vi "Stages Messenger limit check.vi"(0 "Stage Notifier Name":string="ProScan3", 2 "Actions":T2, 5 "Setpoint":dbl[](array[numeric]), 7 "Axis":bool[](array[boolean]), 9 "Velocity":dbl, 11 "Misc":variant, 13 "Exit While Busy?":bool) -> (4 "Stage Notifier Name (Dup)":string, 6 "Positions":dbl[](array[numeric]), 8 "Status":T1, 15 "Error":errorcluster)   [LabVIEW 2021]
uses:
  Stages Controls/Stage Actions.ctl
  Stages Controls/Stage Status.ctl
  Stages Controls/Stage Notifier Element.ctl
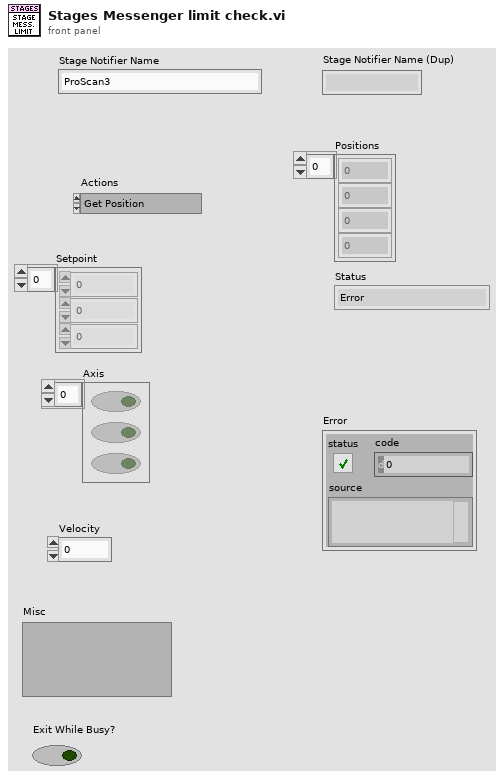
[diagram p1: front panel]
types:
  T1 = typedef "Stage Status.ctl" = enum16{"Error", "Abort", "Busy", "On Target"}
  T2 = typedef "Stage Actions.ctl" = enum16{"Get Position", "SERVO OFF", "SERVO ON", "SERVO ON/OFF", "MVR", "MOVE", "HALT", "ONTARGET", "ERROR", "REFERENCE", "INIT", "VELOCITY", "STATUS", "EXIT", "HOME", "ZEROPOS", "NANOPOS", "ANALOG", "QUIT"}
  T3 = typedef "Stage Notifier Element.ctl" = cluster{"Action":T2, "Axis":bool[], "Setpoint":dbl[], "Velocity":dbl, "Cmd Recvd?":bool, "Position":dbl[], "Status":T1, "Misc":variant, "Servo On?":bool}
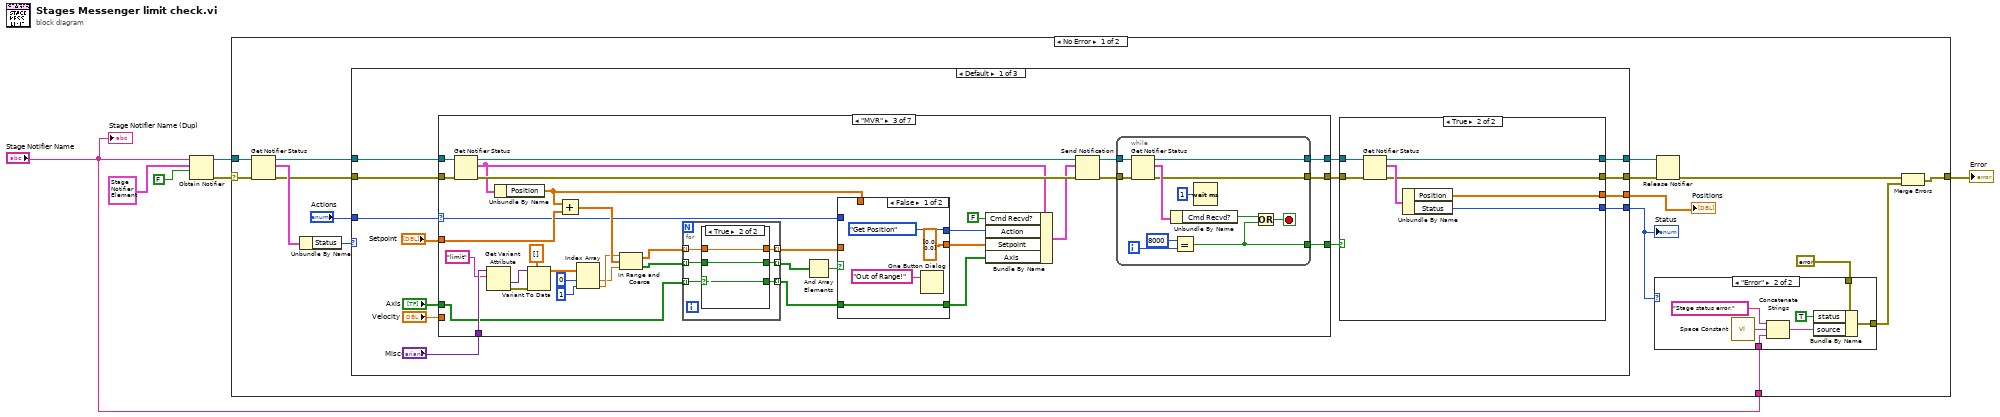
[diagram p0: block diagram]
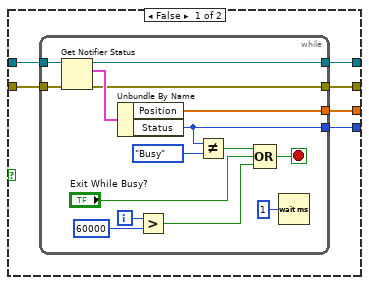
[diagram p3: hidden frame]
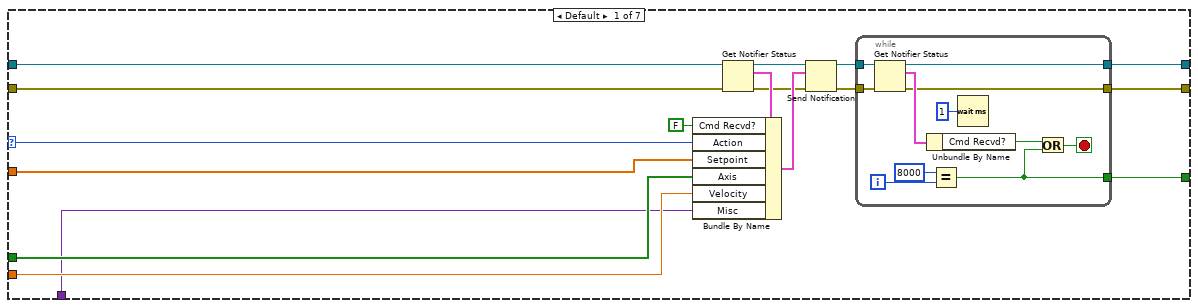
[diagram p4: hidden frame]
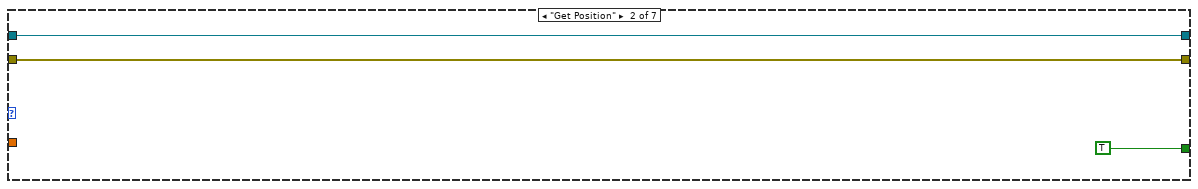
[diagram p5: hidden frame]
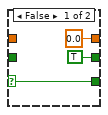
[diagram p6: hidden frame]
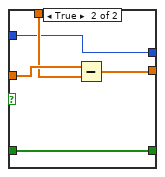
[diagram p7: hidden frame]
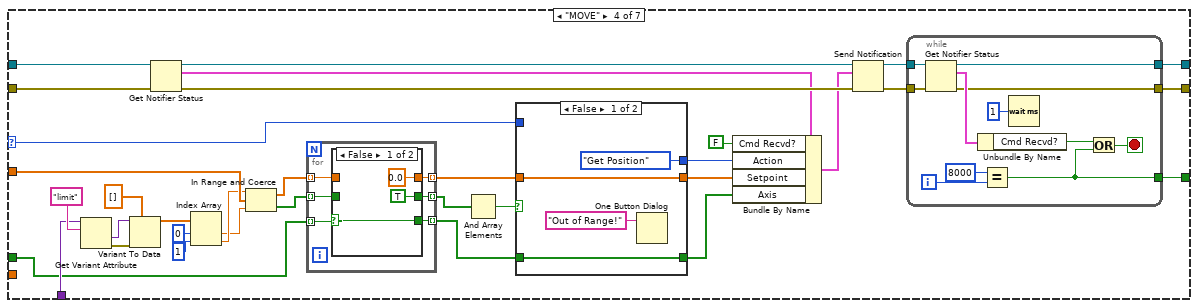
[diagram p8: hidden frame]
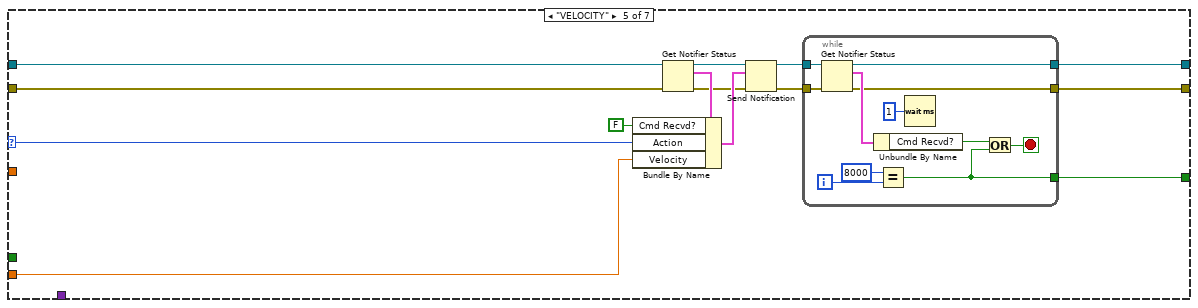
[diagram p11: hidden frame]
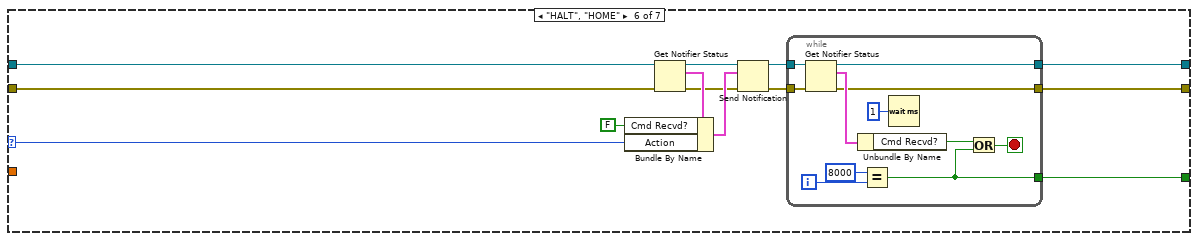
[diagram p12: hidden frame]
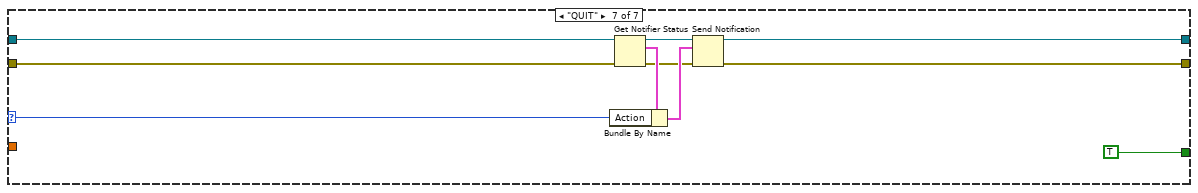
[diagram p13: hidden frame]
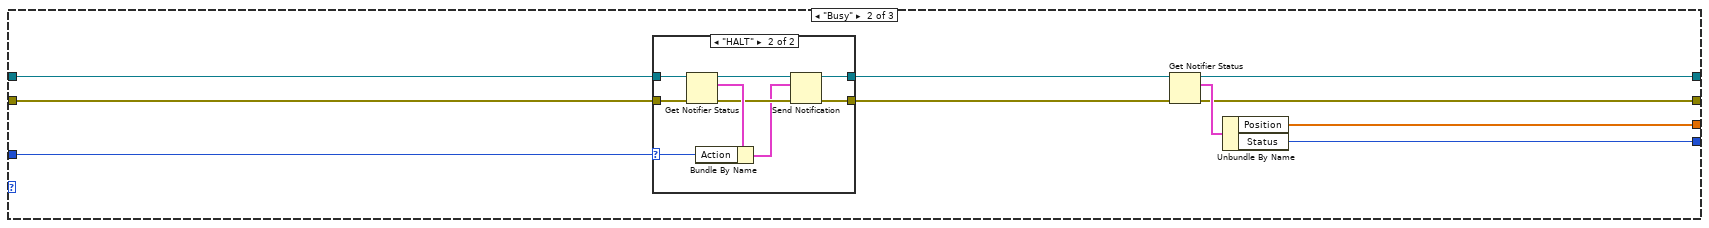
[diagram p14: hidden frame]
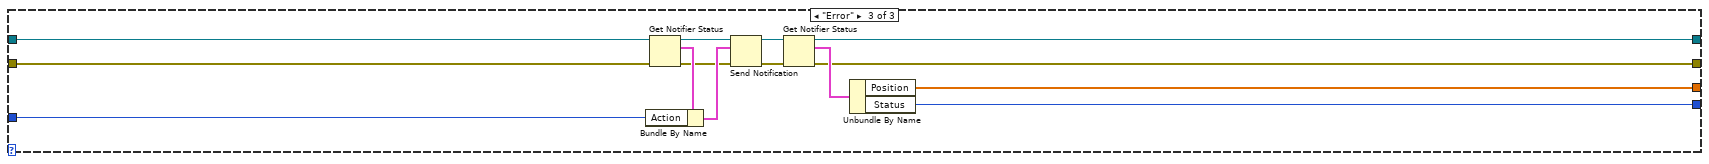
[diagram p16: hidden frame]
diagram:
  n1 = Obtain Notifier(name (unnamed)="Stage Notifier Name", notification data type=T3 {"Action"=enum."Get Position", "Axis"=[], "Setpoint"=[], "Velocity"=0.5, "Cmd Recvd?"=FALSE, "Position"=[], "Status"=enum."Error", "Misc"=variant, "Servo On?"=FALSE} ("Stage Status"), create if not found? (T)=FALSE) -> (notifier out=w3:refnum<notifier>, error out=w4:errorcluster)  [unwired: 1 in, 1 out]
  n2 = case shown="No Error" w4 {
    selector: w4 -> [w16 w330]
    tunnel: w3 -> [w22 _]
    tunnel: "Stage Notifier Name" -> [w11 _]
    tunnel: [w8 w330] -> w1
    frame No Error {
      n3 = Get Notifier Status(notifier=w22, error in (no error)=w16) -> (notifier out=w20:refnum<notifier>, current notification=w21:T3, error out=w15:errorcluster)  [unwired: 2 out]
      n4 = Unbundle By Name(w21) -> ("Status"=w13:T1)
      n5 = case shown="Default" w13 {
        tunnel: w20 -> [w44 w298 w329]
        tunnel: [w37 w303 w323] -> w19
        tunnel: [w36 w302 w322] -> w18
        tunnel: [w35 w301 w321] -> w12
        tunnel: "Actions" -> [w43 w299 w327]
        tunnel: w15 -> [w34 w297 w319]
        tunnel: [w32 w300 w316] -> w14
        frame Default {
          n6 = case shown="\"MVR\"" w43 {
            selector: w43 -> [w85 _ w112 w180 w245 w269 w290]
            tunnel: w44 -> [w86 w103 w138 w204 w246 w270 w293]
            tunnel: [w79 w103 w135 w201 w242 w266 w294] -> w38
            tunnel: "Setpoint" -> [w82 _ w126 w191 _ _ _]
            tunnel: "Axis" -> [w81 _ w109 w178 _ _ _]
            tunnel: "Velocity" -> [w80 _ _ _ w236 _ _]
            tunnel: "Misc" -> [w73 _ w122 w185 _ _ _]
            tunnel: [w78 TRUE w134 w200 w241 w265 TRUE] -> w39
            tunnel: w34 -> [w77 w102 w133 w199 w240 w264 w287]
            tunnel: [w74 w102 w130 w196 w237 w261 w285] -> w33
            frame Default {
              n7 = Get Notifier Status(notifier=w86, error in (no error)=w77) -> (notifier out=w87:refnum<notifier>, current notification=w88:T3, error out=w76:errorcluster)  [unwired: 2 out]
              n8 = Bundle By Name(cluster=w88, "Cmd Recvd?"=FALSE, "Action"=w85, "Setpoint"=w82, "Axis"=w81, "Velocity"=w80, "Misc"=w73) -> (w89:T3)
              n9 = Send Notification(notification=w89, notifier=w87, error in (no error)=w76) -> (notifier out=w83:refnum<notifier>, error out=w75:errorcluster)
              n10 = while {
                tunnel: w83 -> [w100]
                tunnel: [w97] -> w79
                tunnel: [w93] -> w78
                tunnel: w75 -> [w91]
                tunnel: [w90] -> w74
                i -> [w96]
                stop <- w92 stop-if-true
                n11 = Get Notifier Status(notifier=w100, error in (no error)=w91) -> (notifier out=w97:refnum<notifier>, current notification=w99:T3, error out=w90:errorcluster)  [unwired: 2 out]
                n12 = Unbundle By Name(w99) -> ("Cmd Recvd?"=w94:bool)
                n13 = Equal?(x=8000, y=w96) -> (x = y?=w93:bool)
                n14 = Wait (ms)(milliseconds to wait=u32 1) -> ()  [unwired: 1 out]
                n15 = Or(x=w94, y=w93) -> (x .or. y?=w92:bool)
              }
            }
            frame "Get Position" {
            }
            frame "MVR" {
              n16 = Get Notifier Status(notifier=w138, error in (no error)=w133) -> (notifier out=w139:refnum<notifier>, current notification=w123:T3, error out=w132:errorcluster)  [unwired: 2 out]
              n17 = Get Variant Attribute(Variant=w122, name="limit") -> (value=w113:variant, error out=w120:errorcluster)  [unwired: 2 in, 2 out]
              n18 = Unbundle By Name(w123) -> ("Position"=w128:dbl[])
              n19 = Variant To Data(error in=w120, type=dbl[] [] ("Array"), Variant=w113) -> (data=w118:dbl[])  [unwired: 1 out]
              n20 = Add(x=w128, y=w126) -> (x+y=w129:dbl[])
              n21 = Index Array(array=w118, index #1=0 ("index"), index #2=1 ("index")) -> (element #1=w114:dbl, element #2=w115:dbl)
              n22 = In Range and Coerce(upper limit=w115, x=w129, lower limit=w114) -> (coerced(x)=w108:dbl[], In Range?=w107:bool[])
              n23 = for {
                tunnel: w109 -> [w145] mode=indexing
                tunnel: w108 -> [w144] mode=indexing
                tunnel: w107 -> [w143] mode=indexing
                tunnel: [w142] -> w105 mode=indexing
                tunnel: [w141] -> w104 mode=indexing
                tunnel: [w140] -> w110 mode=indexing
                n24 = case shown="True" w145 {
                  selector: w145 -> [w146 w149]
                  tunnel: w144 -> [_ w150]
                  tunnel: w143 -> [_ w151]
                  tunnel: [TRUE ("Position") w151] -> w140
                  tunnel: [0.0 ("Position") w150] -> w142
                  tunnel: [w146 w149] -> w141
                  frame False {
                  }
                  frame True {
                  }
                }
              }
              n25 = And Array Elements(Boolean array=w110) -> (logical AND=w106:bool)
              n26 = case shown="False" w106 {
                tunnel: w105 -> [_ w160]
                tunnel: w128 -> [_ w159]
                tunnel: [dbl[] [0.0, 0.0] w158] -> w127
                tunnel: [w154 w157] -> w125
                tunnel: w104 -> [w154 w157]
                tunnel: w112 -> [_ w156]
                tunnel: [Stage_Actions."Get Position" ("Actions") w156] -> w111
                frame False {
                  n27 = One Button Dialog(message="Out of Range!") -> ()  [unwired: 1 in, 1 out]
                }
                frame True {
                  n28 = Subtract(x=w160, y=w159) -> (x-y=w158:dbl[])
                }
              }
              n29 = Bundle By Name(cluster=w123, "Cmd Recvd?"=FALSE, "Action"=w111, "Setpoint"=w127, "Axis"=w125) -> (w124:T3)
              n30 = Send Notification(notification=w124, notifier=w139, error in (no error)=w132) -> (notifier out=w136:refnum<notifier>, error out=w131:errorcluster)
              n31 = while {
                tunnel: w136 -> [w171]
                tunnel: [w168] -> w135
                tunnel: [w164] -> w134
                tunnel: w131 -> [w162]
                tunnel: [w161] -> w130
                i -> [w167]
                stop <- w163 stop-if-true
                n32 = Get Notifier Status(notifier=w171, error in (no error)=w162) -> (notifier out=w168:refnum<notifier>, current notification=w170:T3, error out=w161:errorcluster)  [unwired: 2 out]
                n33 = Unbundle By Name(w170) -> ("Cmd Recvd?"=w165:bool)
                n34 = Equal?(x=8000, y=w167) -> (x = y?=w164:bool)
                n35 = Wait (ms)(milliseconds to wait=u32 1) -> ()  [unwired: 1 out]
                n36 = Or(x=w165, y=w164) -> (x .or. y?=w163:bool)
              }
            }
            frame "MOVE" {
              n37 = Get Variant Attribute(Variant=w185, name="limit") -> (value=w181:variant, error out=w189:errorcluster)  [unwired: 2 in, 2 out]
              n38 = Variant To Data(error in=w189, type=dbl[] [] ("Array"), Variant=w181) -> (data=w188:dbl[])  [unwired: 1 out]
              n39 = Get Notifier Status(notifier=w204, error in (no error)=w199) -> (notifier out=w205:refnum<notifier>, current notification=w192:T3, error out=w198:errorcluster)  [unwired: 2 out]
              n40 = Index Array(array=w188, index #1=0 ("index"), index #2=1 ("index")) -> (element #1=w182:dbl, element #2=w183:dbl)
              n41 = In Range and Coerce(upper limit=w183, x=w191, lower limit=w182) -> (coerced(x)=w177:dbl[], In Range?=w176:bool[])
              n42 = for {
                tunnel: w178 -> [w211] mode=indexing
                tunnel: w177 -> [w210] mode=indexing
                tunnel: w176 -> [w209] mode=indexing
                tunnel: [w208] -> w175 mode=indexing
                tunnel: [w207] -> w174 mode=indexing
                tunnel: [w206] -> w172 mode=indexing
                n43 = case shown="False" w211 {
                  selector: w211 -> [w212 w215]
                  tunnel: w210 -> [_ w216]
                  tunnel: w209 -> [_ w217]
                  tunnel: [TRUE ("Position") w217] -> w206
                  tunnel: [0.0 ("Position") w216] -> w208
                  tunnel: [w212 w215] -> w207
                  frame False {
                  }
                  frame True {
                  }
                }
              }
              n44 = And Array Elements(Boolean array=w172) -> (logical AND=w173:bool)
              n45 = case shown="False" w173 {
                tunnel: w175 -> [w220 w223]
                tunnel: [w220 w223] -> w195
                tunnel: [w218 w224] -> w194
                tunnel: w174 -> [w218 w224]
                tunnel: w180 -> [_ w222]
                tunnel: [Stage_Actions."Get Position" ("Actions") w222] -> w179
                frame False {
                  n46 = One Button Dialog(message="Out of Range!") -> ()  [unwired: 1 in, 1 out]
                }
                frame True {
                }
              }
              n47 = Bundle By Name(cluster=w192, "Cmd Recvd?"=FALSE, "Action"=w179, "Setpoint"=w195, "Axis"=w194) -> (w193:T3)
              n48 = Send Notification(notification=w193, notifier=w205, error in (no error)=w198) -> (notifier out=w202:refnum<notifier>, error out=w197:errorcluster)
              n49 = while {
                tunnel: w202 -> [w235]
                tunnel: [w232] -> w201
                tunnel: [w228] -> w200
                tunnel: w197 -> [w226]
                tunnel: [w225] -> w196
                i -> [w231]
                stop <- w227 stop-if-true
                n50 = Get Notifier Status(notifier=w235, error in (no error)=w226) -> (notifier out=w232:refnum<notifier>, current notification=w234:T3, error out=w225:errorcluster)  [unwired: 2 out]
                n51 = Unbundle By Name(w234) -> ("Cmd Recvd?"=w229:bool)
                n52 = Equal?(x=8000, y=w231) -> (x = y?=w228:bool)
                n53 = Wait (ms)(milliseconds to wait=u32 1) -> ()  [unwired: 1 out]
                n54 = Or(x=w229, y=w228) -> (x .or. y?=w227:bool)
              }
            }
            frame "VELOCITY" {
              n55 = Get Notifier Status(notifier=w246, error in (no error)=w240) -> (notifier out=w247:refnum<notifier>, current notification=w248:T3, error out=w239:errorcluster)  [unwired: 2 out]
              n56 = Bundle By Name(cluster=w248, "Cmd Recvd?"=FALSE, "Action"=w245, "Velocity"=w236) -> (w249:T3)
              n57 = Send Notification(notification=w249, notifier=w247, error in (no error)=w239) -> (notifier out=w243:refnum<notifier>, error out=w238:errorcluster)
              n58 = while {
                tunnel: w243 -> [w260]
                tunnel: [w257] -> w242
                tunnel: [w253] -> w241
                tunnel: w238 -> [w251]
                tunnel: [w250] -> w237
                i -> [w256]
                stop <- w252 stop-if-true
                n59 = Get Notifier Status(notifier=w260, error in (no error)=w251) -> (notifier out=w257:refnum<notifier>, current notification=w259:T3, error out=w250:errorcluster)  [unwired: 2 out]
                n60 = Unbundle By Name(w259) -> ("Cmd Recvd?"=w254:bool)
                n61 = Equal?(x=8000, y=w256) -> (x = y?=w253:bool)
                n62 = Wait (ms)(milliseconds to wait=u32 1) -> ()  [unwired: 1 out]
                n63 = Or(x=w254, y=w253) -> (x .or. y?=w252:bool)
              }
            }
            frame "HALT", "HOME" {
              n64 = Get Notifier Status(notifier=w270, error in (no error)=w264) -> (notifier out=w271:refnum<notifier>, current notification=w272:T3, error out=w263:errorcluster)  [unwired: 2 out]
              n65 = Bundle By Name(cluster=w272, "Cmd Recvd?"=FALSE, "Action"=w269) -> (w273:T3)
              n66 = Send Notification(notification=w273, notifier=w271, error in (no error)=w263) -> (notifier out=w267:refnum<notifier>, error out=w262:errorcluster)
              n67 = while {
                tunnel: w267 -> [w284]
                tunnel: [w281] -> w266
                tunnel: [w277] -> w265
                tunnel: w262 -> [w275]
                tunnel: [w274] -> w261
                i -> [w280]
                stop <- w276 stop-if-true
                n68 = Get Notifier Status(notifier=w284, error in (no error)=w275) -> (notifier out=w281:refnum<notifier>, current notification=w283:T3, error out=w274:errorcluster)  [unwired: 2 out]
                n69 = Unbundle By Name(w283) -> ("Cmd Recvd?"=w278:bool)
                n70 = Equal?(x=8000, y=w280) -> (x = y?=w277:bool)
                n71 = Wait (ms)(milliseconds to wait=u32 1) -> ()  [unwired: 1 out]
                n72 = Or(x=w278, y=w277) -> (x .or. y?=w276:bool)
              }
            }
            frame "QUIT" {
              n73 = Get Notifier Status(notifier=w293, error in (no error)=w287) -> (notifier out=w292:refnum<notifier>, current notification=w291:T3, error out=w286:errorcluster)  [unwired: 2 out]
              n74 = Bundle By Name(cluster=w291, "Action"=w290) -> (w289:T3)
              n75 = Send Notification(notification=w289, notifier=w292, error in (no error)=w286) -> (notifier out=w294:refnum<notifier>, error out=w285:errorcluster)
            }
          }
          n76 = case shown="True" w39 {
            tunnel: w38 -> [w50 w72]
            tunnel: [w49 w71] -> w37
            tunnel: [w48 w70] -> w36
            tunnel: [w47 w68] -> w35
            tunnel: w33 -> [w46 w67]
            tunnel: [w45 w66] -> w32
            frame False {
              n77 = while {
                tunnel: w50 -> [w65]
                tunnel: [w64] -> w49
                tunnel: [w62] -> w48
                tunnel: [w56] -> w47
                tunnel: w46 -> [w52]
                tunnel: [w51] -> w45
                i -> [w58]
                stop <- w53 stop-if-true
                n78 = Get Notifier Status(notifier=w65, error in (no error)=w52) -> (notifier out=w64:refnum<notifier>, current notification=w63:T3, error out=w51:errorcluster)  [unwired: 2 out]
                n79 = Unbundle By Name(w63) -> ("Position"=w62:dbl[], "Status"=w56:T1)
                n80 = Greater?(x=w58, y=60000) -> (0:w54:bool)
                n81 = Not Equal?(x=w56, y=Stage_Status."Busy") -> (x != y?=w59:bool)
                n82 = Compound Arithmetic op=OR(w59, "Exit While Busy?", w54) -> (w53:bool)
                n83 = Wait (ms)(milliseconds to wait=u32 1) -> ()  [unwired: 1 out]
              }
            }
            frame True {
              n84 = Get Notifier Status(notifier=w72, error in (no error)=w67) -> (notifier out=w71:refnum<notifier>, current notification=w69:T3, error out=w66:errorcluster)  [unwired: 2 out]
              n85 = Unbundle By Name(w69) -> ("Position"=w70:dbl[], "Status"=w68:T1)
            }
          }
        }
        frame "Busy" {
          n86 = case shown="\"HALT\"" w299 {
            selector: w299 -> [_ w312]
            tunnel: w298 -> [w306 w315]
            tunnel: w297 -> [w305 w314]
            tunnel: [w306 w309] -> w296
            tunnel: [w305 w308] -> w295
            frame Default {
            }
            frame "HALT" {
              n87 = Get Notifier Status(notifier=w315, error in (no error)=w314) -> (notifier out=w311:refnum<notifier>, current notification=w313:T3, error out=w310:errorcluster)  [unwired: 2 out]
              n88 = Bundle By Name(cluster=w313, "Action"=w312) -> (w307:T3)
              n89 = Send Notification(notification=w307, notifier=w311, error in (no error)=w310) -> (notifier out=w309:refnum<notifier>, error out=w308:errorcluster)
            }
          }
          n90 = Get Notifier Status(notifier=w296, error in (no error)=w295) -> (notifier out=w303:refnum<notifier>, current notification=w304:T3, error out=w300:errorcluster)  [unwired: 2 out]
          n91 = Unbundle By Name(w304) -> ("Position"=w302:dbl[], "Status"=w301:T1)
        }
        frame "Error" {
          n92 = Get Notifier Status(notifier=w329, error in (no error)=w319) -> (notifier out=w326:refnum<notifier>, current notification=w328:T3, error out=w318:errorcluster)  [unwired: 2 out]
          n93 = Bundle By Name(cluster=w328, "Action"=w327) -> (w325:T3)
          n94 = Send Notification(notification=w325, notifier=w326, error in (no error)=w318) -> (notifier out=w324:refnum<notifier>, error out=w317:errorcluster)
          n95 = Get Notifier Status(notifier=w324, error in (no error)=w317) -> (notifier out=w323:refnum<notifier>, current notification=w320:T3, error out=w316:errorcluster)  [unwired: 2 out]
          n96 = Unbundle By Name(w320) -> ("Position"=w322:dbl[], "Status"=w321:T1)
        }
      }
      "Positions" <- w18
      "Status" <- w12
      n97 = case shown="\"Error\"" w12 {
        tunnel: w11 -> [_ w27]
        tunnel: [w23 w25] -> w9
        tunnel: errorcluster {"status"=FALSE, "code"=0, "source"=""} ("Error 2") -> [w23 w24]
        frame Default {
        }
        frame "Error" {
          n98 = call <vilib>:"Space Constant.vi"() -> ("String"=w28:string)
          n99 = Concatenate Strings("Stage status error." ("source"), w28, w27) -> (w26:string)
          n100 = Bundle By Name(cluster=w24, "status"=TRUE, "source"=w26) -> (w25:errorcluster)
        }
      }
      n101 = Release Notifier(notifier=w19, error in (no error)=w14) -> (error out=w10:errorcluster)  [unwired: 1 in, 2 out]
      n102 = Merge Errors(w10, w9) -> (w8:errorcluster)
    }
    frame Error {
    }
  }
  "Error" <- w1
  "Stage Notifier Name (Dup)" <- "Stage Notifier Name"
